vi "Init.vi"(8 "error in (no error)":errorcluster, 11 "VISA resource name":refnum<visa-resource-name>) -> (0 "error out":errorcluster, 3 "VISA resource name out":refnum<visa-resource-name>)   [LabVIEW 2011, in "Magna PSU.lvlib"]
uses:
  Magna PSU.lvlib
  <vilib>/Instr/_visa.llb/VISA Configure Serial Port (Instr).vi
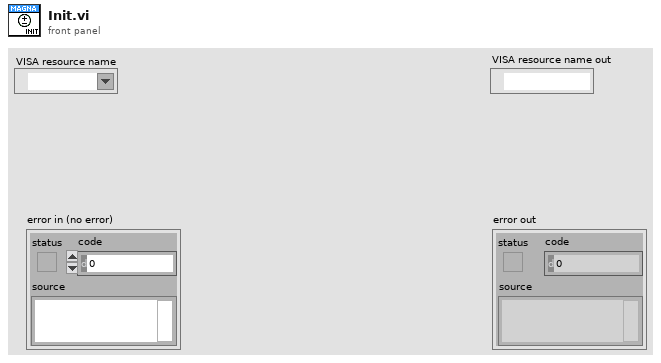
[diagram p1: front panel]
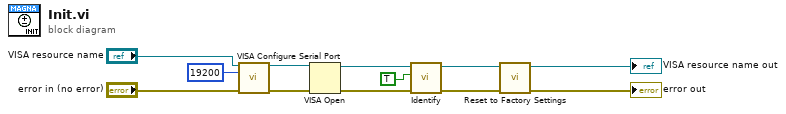
[diagram p0: block diagram]
diagram:
  n1 = call-poly "VISA Configure Serial Port"("VISA resource name"="VISA resource name", "baud rate (9600)"=u32 19200, "error in (no error)"="error in (no error)") -> ("VISA resource name out"=w9:refnum<visa-resource-name>, "error out"=w8:errorcluster)  [unwired: 11 in]
  n2 = VISA Open(error in (no error)=w8, VISA resource name=w9) -> (VISA resource name=w7:refnum<visa-resource-name>, error out=w6:errorcluster)  [unwired: 3 in]
  n3 = call "Identify.vi"("error in (no error)"=w6, "Write IDN"=TRUE, "VISA Refnum in"=w7) -> ("error out"=w4:errorcluster, "VISA Refnum out"=w3:refnum<visa-resource-name>)  [unwired: 7 in]
  n4 = call "Reset to Factory Settings.vi"("error in (no error)"=w4, "VISA Refnum in"=w3) -> ("error out"=→"error out":errorcluster, "VISA Refnum out"=→"VISA resource name out":refnum<visa-resource-name>)  [unwired: 8 in]
